vi "TCP Generic Grab Data.vi"(0 "connection ID":refnum<k5>, 7 "No timeout?":bool, 9 "byte order":T1(ring)=enum."native, host order", 11 "error in (no error)":errorcluster) -> (4 "connection ID out":refnum<k5>, 6 "data out":string, 15 "error out":errorcluster)   [LabVIEW 2020]
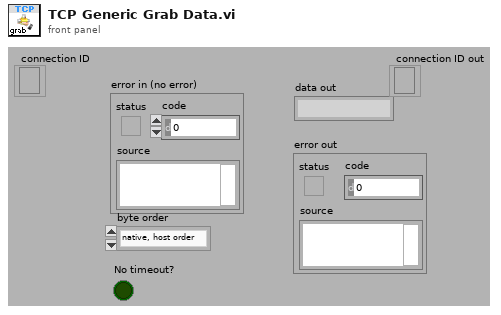
[diagram p1: front panel]
types:
  T1 = enum16{"big-endian, network order", "native, host order", "little-endian"}
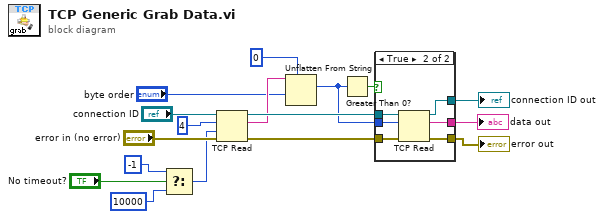
[diagram p0: block diagram]
diagram:
  n1 = Select(t=-1 ("timeout ms (25000)"), s="No timeout?", f=10000 ("timeout ms (25000)")) -> (s? t:f=w9:i32)
  n2 = TCP Read(connection ID="connection ID", bytes to read=4, error in (no error)="error in (no error)", 9:w9) -> (connection ID out=w14:refnum<k5>, data out=w5:string, error out=w13:errorcluster)  [unwired: 1 in]
  n3 = Unflatten From String(type=0, binary string=w5, byte order (0:big-endian, network order)="byte order") -> (value=w1:i32)  [unwired: 2 in, 2 out]
  n4 = Greater Than 0?(x=w1) -> (x > 0?=w12:bool)
  n5 = case shown="True" w12 {
    tunnel: [_ w25] -> w17
    tunnel: [w19 w24] -> w16
    tunnel: w14 -> [w18 w23]
    tunnel: w13 -> [w19 w22]
    tunnel: w1 -> [_ w21]
    tunnel: [w18 w20] -> w6
    frame False {
    }
    frame True {
      n6 = TCP Read(connection ID=w23, bytes to read=w21, error in (no error)=w22) -> (connection ID out=w20:refnum<k5>, data out=w25:string, error out=w24:errorcluster)  [unwired: 2 in]
    }
  }
  "data out" <- w17
  "error out" <- w16
  "connection ID out" <- w6
